vi "B-Scan (LLC messages).vi"(7 "Micropulse # In":i32, 9 "Scan definition":T1={"Scan Start"=0.0, "Scan Length"=280.0, "Inspection Resolution"=0.5, "Direction"=enum."Forwards"} {"Inspection Resolution" format="%#_6f"; "Scan Start" format="%#_6f"; "Scan Length" format="%#_6f"}, 10 "Axis No.":u8=1 min=1 max=4, 11 "scan data info":T3 {"Error Message" format="%04x"; "Message Header" format="%04x"; "IP"."MIP location" format="%#.0f"; "IP"."Location" format="%#.0f"; "PRF" format="%.0fHz"}) -> (0 "Update Display?":bool, 1 "B-Scan In Progress?":bool, 2 "B-Scan index":i32, 3 "B-Scan Out":u16[][](array[numeric]))   [LabVIEW 2026, in "MicroPulse_Driver.lvlib"]
uses:
  MicroPulse_Driver.lvlib
  Data/Datatypes/MP - scan data info.ctl
  Data/Datatypes/MP - data output format.ctl
  Data/Datatypes/MP - retain scan.ctl
  Data/Datatypes/MP - axis positions (LLC).ctl
  Data/Datatypes/MP - fly scan range.ctl
  Data/Datatypes/MP - inspection direction.ctl
  Low Level/FGV - B-Scan Active - Action [Enum].ctl
  <instrlib>/Micropulse/Micropulse.lvlib
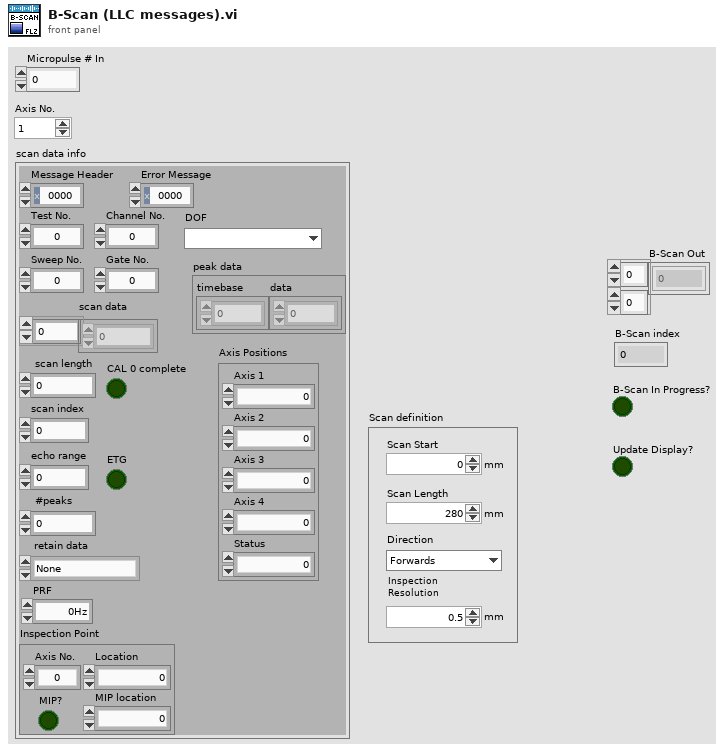
[diagram p1: front panel]
types:
  T1 = typedef "Micropulse.lvlib/MP - fly scan range.ctl" = cluster{"Scan Start":dbl, "Scan Length":dbl, "Inspection Resolution":dbl, "Direction":T2}
  T2 = typedef "Micropulse.lvlib/MP - inspection direction.ctl" = enum16{"Forwards", "Backwards"}
  T3 = typedef "Micropulse.lvlib/MP - scan data info.ctl" = cluster{"Message Header":u16, "Error Message":u16, "Test No.":u32, "Channel No.":u8, "Sweep No.":u32, "Gate No.":u32, "DOF":T4, "retain data":T5, "scan data":u16[], "scan length":i32, "scan index":i32, "peak data":cluster{"timebase":u16[], "data":u16[]}, "#peaks":i32, "PRF":dbl, "IP":cluster{"Axis No.":u8, "Location":u32, "MIP location":u32, "MIP?":bool}, "echo range":u16, "ETG":bool, "CAL 0 complete":bool, "Axis Positions":T6}
  T4 = typedef "Micropulse.lvlib/MP - data output format.ctl" = enum16{"", "8-bit Mode", "10-bit Mode", "12-bit Mode", "16-bit Mode", "8-bit Log Mode", "12-bit Packed Mode"}
  T5 = typedef "Micropulse.lvlib/MP - retain scan.ctl" = enum16{"None", "Ascan", "Peaks"}
  T6 = typedef "Micropulse.lvlib/MP - axis positions (LLC).ctl" = cluster{"Axis 1":u32, "Axis 2":u32, "Axis 3":u32, "Axis 4":u32, "Status":u8}
  T7 = typedef "MicroPulse_Driver.lvlib/FGV - B-Scan Active - Action [Enum].ctl" = enum16{"Read", "Read & Reset Start Flag", "Start B-Scan", "B-Scan Finished"}
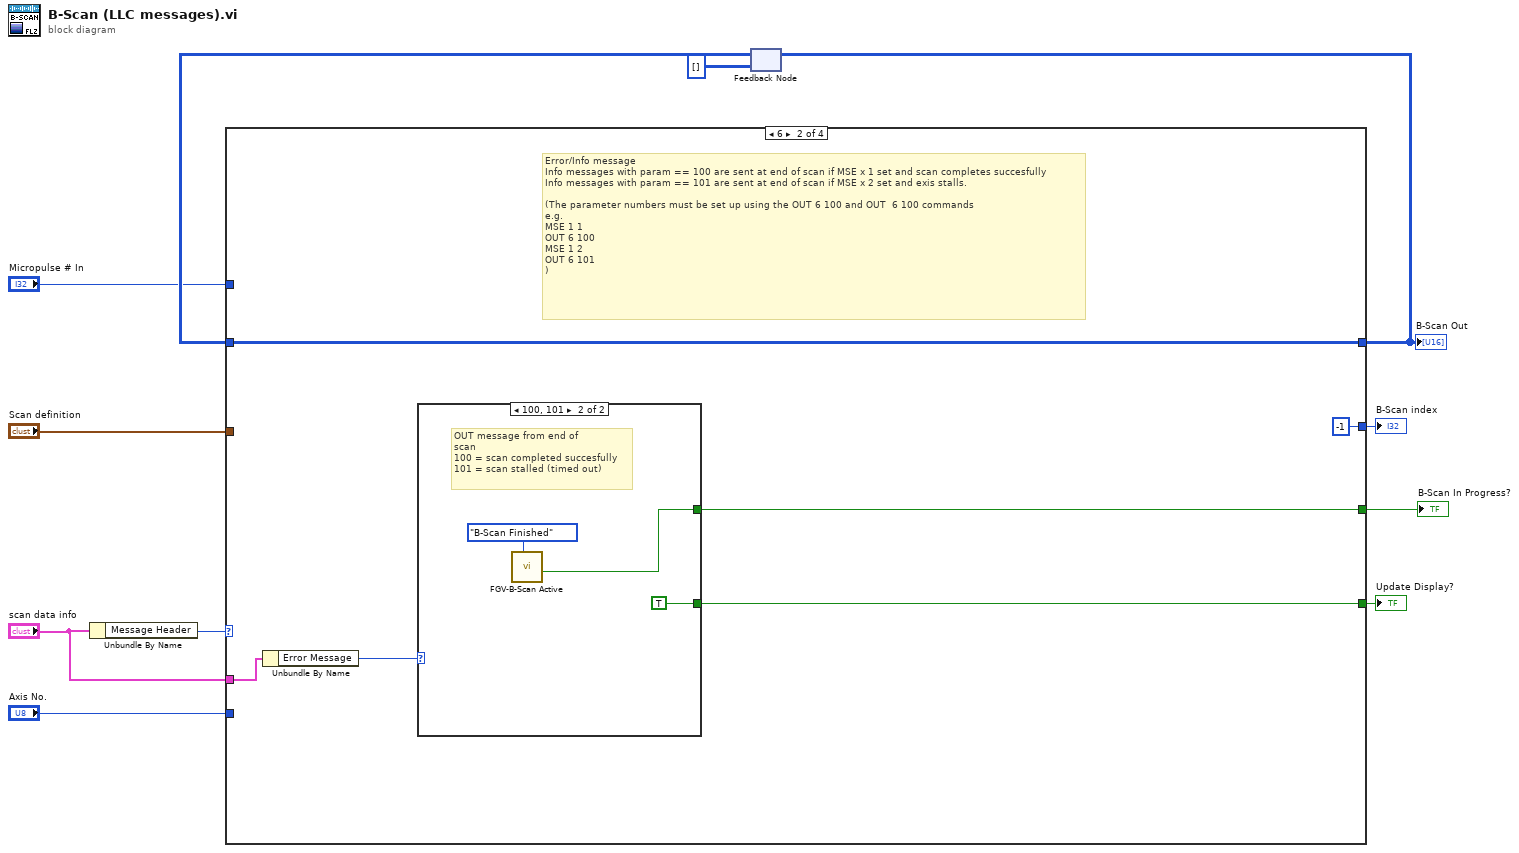
[diagram p0: block diagram]
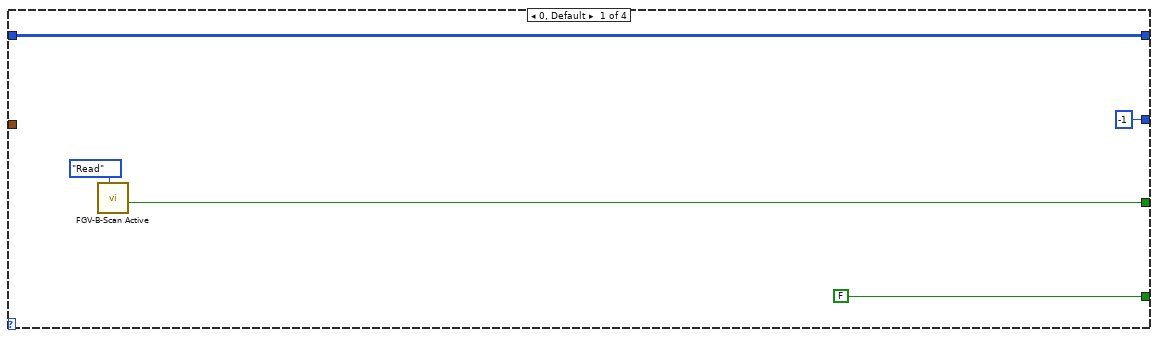
[diagram p2: hidden frame]
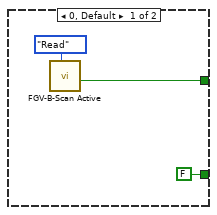
[diagram p3: hidden frame]
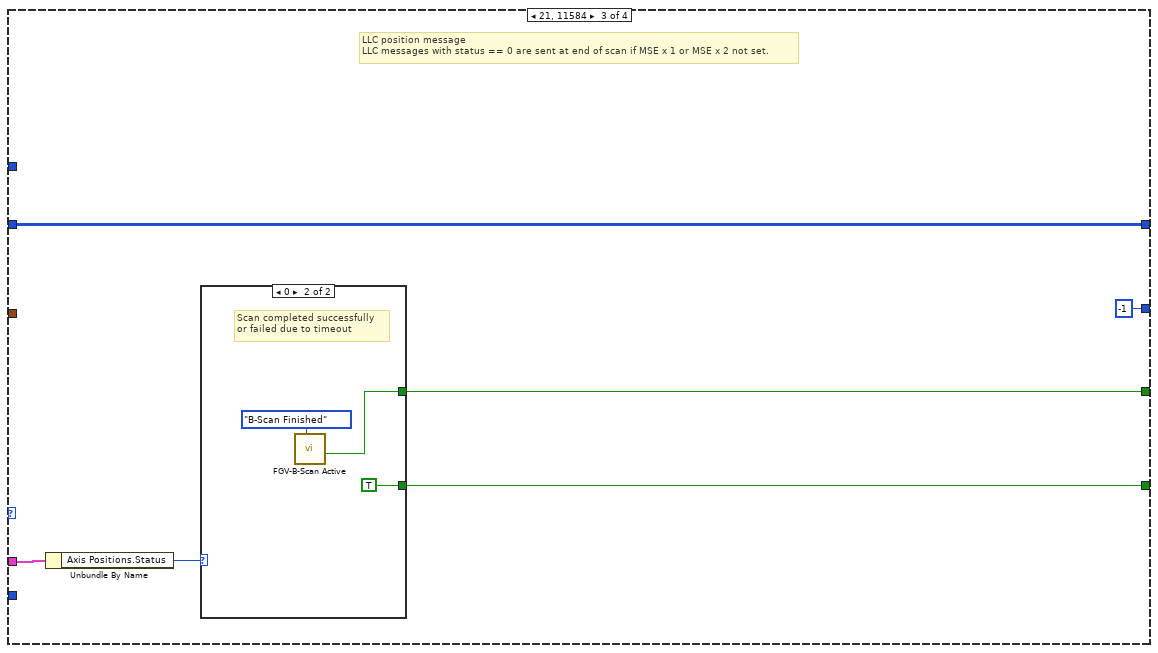
[diagram p4: hidden frame]
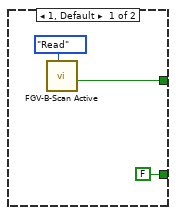
[diagram p5: hidden frame]
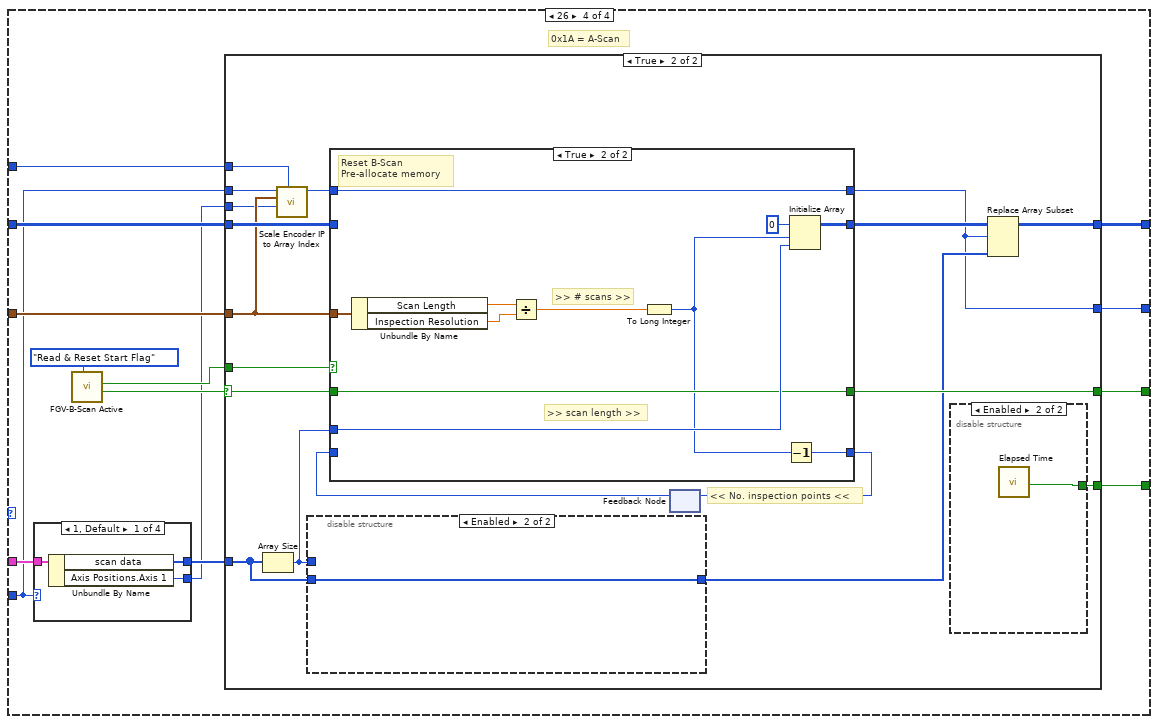
[diagram p6: hidden frame]
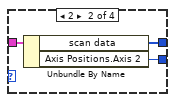
[diagram p7: hidden frame]
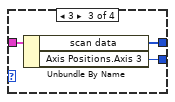
[diagram p8: hidden frame]
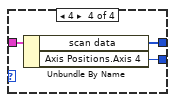
[diagram p9: hidden frame]
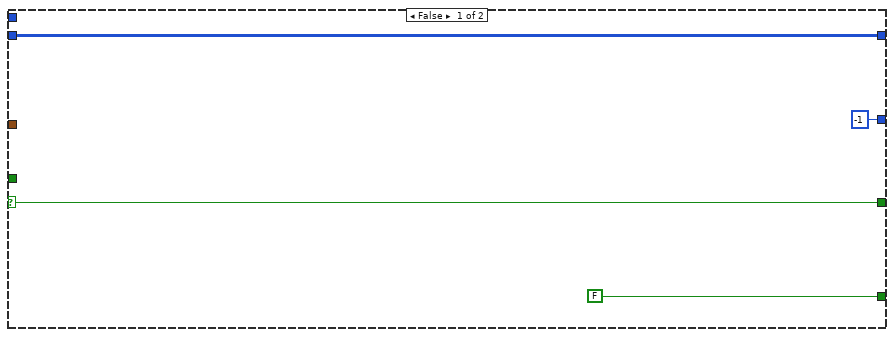
[diagram p10: hidden frame]
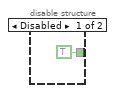
[diagram p11: hidden frame]
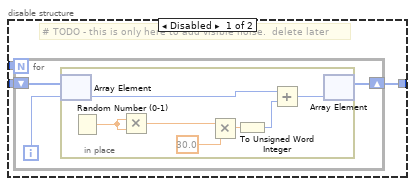
[diagram p12: hidden frame]
diagram:
  n1 = Unbundle By Name("scan data info") -> ("Message Header"=w11:u16)
  n2 = feedback #1(u16[][] []) -> (w7:u16[][])
  n3 = case shown="6" w11 {
    tunnel: "scan data info" -> [_ w21 w33 w54]
    tunnel: "Scan definition" -> [_ _ _ w48]
    tunnel: [w16 w22 w34 w52] -> w8
    tunnel: w7 -> [w16 w22 w34 w51]
    tunnel: "Micropulse # In" -> [_ _ _ w47]
    tunnel: [w13 w19 w31 w50] -> w4
    tunnel: [FALSE w17 w29 w49] -> w3
    tunnel: "Axis No." -> [_ _ _ w42]
    tunnel: [-1 ("B-Scan index") -1 ("B-Scan index") -1 ("B-Scan index") w41] -> w1
    frame 0, Default {
      n4 = call "FGV-B-Scan Active.vi"("Action"=FGV_-_B-Scan_Active_-_Action_[Enum]."Read") -> ("B-Scan In Progress?"=w13:bool)  [unwired: 8 in, 2 out]
    }
    frame 6 {
      # "Error/Info message\nInfo messages with param == 100 are sent at end of scan if MSE x 1 set and scan completes succesfully\nInfo messages with param == 101 are sent at end of scan if MSE x 2 set and exis stalls.\n\n(The parameter numbers must be set up using the OUT 6 100 and OUT  6 100 commands \ne.g.\nMSE 1 1\nOUT 6 100\nMSE 1 2\nOUT 6 101\n)"
      n5 = Unbundle By Name(w21) -> ("Error Message"=w20:u16)
      n6 = case shown="100, 101" w20 {
        tunnel: [w24 w27] -> w19
        tunnel: [FALSE TRUE] -> w17
        frame 0, Default {
          n7 = call "FGV-B-Scan Active.vi"("Action"=FGV_-_B-Scan_Active_-_Action_[Enum]."Read") -> ("B-Scan In Progress?"=w24:bool)  [unwired: 8 in, 2 out]
        }
        frame 100, 101 {
          # "OUT message from end of\nscan\n100 = scan completed succesfully\n101 = scan stalled (timed out)"
          n8 = call "FGV-B-Scan Active.vi"("Action"=FGV_-_B-Scan_Active_-_Action_[Enum]."B-Scan Finished") -> ("B-Scan In Progress?"=w27:bool)  [unwired: 8 in, 2 out]
        }
      }
    }
    frame 21, 11584 {
      # "LLC position message\nLLC messages with status == 0 are sent at end of scan if MSE x 1 or MSE x 2 not set."
      n9 = Unbundle By Name(w33) -> ("Axis Positions.Status"=w32:u8)
      n10 = case shown="0" w32 {
        tunnel: [w36 w39] -> w31
        tunnel: [FALSE TRUE] -> w29
        frame 1, Default {
          n11 = call "FGV-B-Scan Active.vi"("Action"=FGV_-_B-Scan_Active_-_Action_[Enum]."Read") -> ("B-Scan In Progress?"=w36:bool)  [unwired: 8 in, 2 out]
        }
        frame 0 {
          # "Scan completed successfully\nor failed due to timeout"
          n12 = call "FGV-B-Scan Active.vi"("Action"=FGV_-_B-Scan_Active_-_Action_[Enum]."B-Scan Finished") -> ("B-Scan In Progress?"=w39:bool)  [unwired: 8 in, 2 out]
        }
      }
    }
    frame 26 {
      # "0x1A = A-Scan"
      n13 = case shown="1, Default" w42 {
        tunnel: w54 -> [w57 w60 w63 w66]
        tunnel: [w56 w59 w62 w65] -> w53
        tunnel: [w55 w58 w61 w64] -> w43
        frame 1, Default {
          n14 = Unbundle By Name(w57) -> ("scan data"=w56:u16[], "Axis Positions.Axis 1"=w55:u32)
        }
        frame 2 {
          n15 = Unbundle By Name(w60) -> ("scan data"=w59:u16[], "Axis Positions.Axis 2"=w58:u32)
        }
        frame 3 {
          n16 = Unbundle By Name(w63) -> ("scan data"=w62:u16[], "Axis Positions.Axis 3"=w61:u32)
        }
        frame 4 {
          n17 = Unbundle By Name(w66) -> ("scan data"=w65:u16[], "Axis Positions.Axis 4"=w64:u32)
        }
      }
      n18 = call "FGV-B-Scan Active.vi"("Action"=FGV_-_B-Scan_Active_-_Action_[Enum]."Read & Reset Start Flag") -> ("B-Scan In Progress?"=w44:bool, "B-Scan Start?"=w45:bool)  [unwired: 8 in, 1 out]
      n19 = case shown="True" w44 {
        selector: w44 -> [w69 w82]
        tunnel: w51 -> [w70 w88]
        tunnel: [w70 w86] -> w52
        tunnel: w53 -> [_ w77]
        tunnel: w48 -> [_ w74]
        tunnel: [w69 w83] -> w50
        tunnel: [FALSE w81] -> w49
        tunnel: w47 -> [_ w78]
        tunnel: w45 -> [_ w75]
        tunnel: w43 -> [_ w73]
        tunnel: w42 -> [_ w72]
        tunnel: [-1 ("B-Scan index") w71] -> w41
        frame False {
        }
        frame True {
          # "<< No. inspection points <<"
          n20 = Array Size(array=w77) -> (size(s)=w76:i32)
          n21 = call "Scale Encoder IP to Array Index.vi"("Micropulse # In"=w78, "Inspection Point Location"=w73, "Scan definition"=w74, "Axis No."=w72) -> ("B-Scan index"=w79:i32)  [unwired: 6 in, 1 out]
          n22 = disable-structure shown="Enabled" {
            disable-tunnel: [w93 w104] -> w80
            disable-tunnel: w77 -> [w92 w104]
            disable-tunnel: w76 -> [w91 _]
            frame Disabled {
              # "# TODO - this is only here to add visible noise.  delete later"
              n23 = for {
                N: w91 -> [_]
                shift-right: [w94] -> w93
                shift-left: w92 -> [w96]
                i -> [w95]
                n24 = in-place {
                  n25 = in-place-array #2(w96, w95) -> (w100:u16)
                  n26 = Random Number (0-1)() -> (number: 0 to 1=w97:dbl)
                  n27 = Multiply(x=w97, y=w97) -> (x*y=w98:dbl)
                  n28 = Multiply(x=w98, y=30.0) -> (x*y=w102:dbl)
                  n29 = To Unsigned Word Integer(number=w102) -> (unsigned 16bit integer=w101:u16)
                  n30 = Add(x=w100, y=w101) -> (x+y=w99:u16)
                  n31 = in-place-array #2(w99) -> (w94:u16[])  [unwired: 1 out]
                }
              }
            }
            frame Enabled {
            }
          }
          n32 = feedback #3() -> (w84:i32)  [unwired: 1 in]
          n33 = case shown="True" w75 {
            tunnel: w88 -> [w108 _]
            tunnel: [w108 w119] -> w87
            tunnel: w74 -> [_ w117]
            tunnel: w76 -> [_ w114]
            tunnel: w79 -> [w106 w110]
            tunnel: [w105 w113] -> w85
            tunnel: w84 -> [w105 _]
            tunnel: [w107 w111] -> w83
            tunnel: w82 -> [w107 w111]
            tunnel: [w106 w110] -> w71
            frame False {
            }
            frame True {
              # "Reset B-Scan\nPre-allocate memory"
              # ">> scan length >>"
              # ">> # scans >>"
              n34 = Unbundle By Name(w117) -> ("Scan Length"=w116:dbl, "Inspection Resolution"=w115:dbl)
              n35 = Divide(x=w116, y=w115) -> (x/y=w112:dbl)
              n36 = To Long Integer(number=w112) -> (32bit integer=w109:i32)
              n37 = Decrement(x=w109) -> (x-1=w113:i32)
              n38 = Initialize Array(u16 0 ("index"), w109, w114) -> (w119:u16[][])
            }
          }
          n39 = feedback-in #3(w85) -> ()
          n40 = disable-structure shown="Enabled" {
            disable-tunnel: [TRUE w90] -> w81
            frame Disabled {
            }
            frame Enabled {
              n41 = call "Elapsed Time"() -> ("Time has Elapsed"=w90:bool)  [unwired: 12 in, 7 out]
            }
          }
          n42 = Replace Array Subset(array=w87, new element=w80, index (row)=w71) -> (w86:u16[][])  [unwired: 1 in]
        }
      }
    }
  }
  "B-Scan Out" <- w8
  "Update Display?" <- w3
  "B-Scan In Progress?" <- w4
  "B-Scan index" <- w1
  n43 = feedback-in #1(w8) -> ()
